vi "Add Common Plugin Properties.vi"(8 "error in":errorcluster, 11 "Clust Refnum":refnum<vi>) -> (0 "error out":errorcluster, 3 "Clust Refnum":refnum<vi>)   [LabVIEW 2026, in "Plugin XML Parser.lvlib"]
uses:
  Plugin XML Parser.lvlib
  <vilib>/numeric/LVNumericRepresentation.ctl
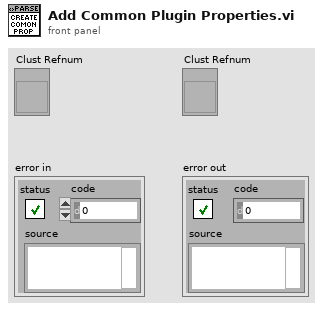
[diagram p1: front panel]
types:
  T1 = typedef "LVNumericRepresentation.ctl" = enum32{"Extended Precision", "Double Precision", "Single Precision", "Long", "Word", "Byte", "Unsigned Long", "Unsigned Word", "Unsigned Byte", "Complex Extended", "Complex Double", "Complex Single", "Quad", "Unsigned Quad", "Fixed-Point"}
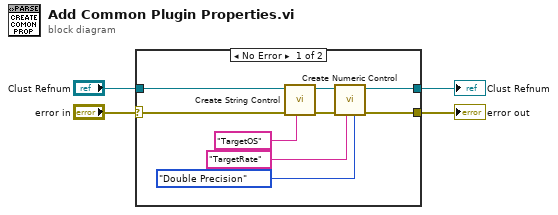
[diagram p0: block diagram]
diagram:
  n1 = case shown="No Error" "error in" {
    selector: "error in" -> [w13 w15]
    tunnel: [w11 w15] -> w3
    tunnel: [w6 w14] -> w2
    tunnel: "Clust Refnum" -> [w10 w14]
    frame No Error {
      n2 = call "Create String Control.vi"("Label.Text"="TargetOS" ("Property Name"), "error in"=w13, "Cluster in"=w10) -> ("error out"=w12:errorcluster, "Cluster out"=w8:refnum<vi>)  [unwired: 7 in]
      n3 = call "Create Numeric Control.vi"("Representation"=LVNumericRepresentation."Double Precision", "Label.Text"="TargetRate" ("Property Name"), "error in"=w12, "Cluster in"=w8) -> ("error out"=w11:errorcluster, "Cluster out"=w6:refnum<vi>)  [unwired: 6 in]
    }
    frame Error {
    }
  }
  "error out" <- w3
  "Clust Refnum" <- w2
